vi "Data Logging Example.vi"() -> ()   [LabVIEW 2016]
panel:
  in  "File Name":string="log1.csv"
  in  "Header String":string="value 1, value 2, value 3"
  out "Line Written":bool=TRUE
  in  "Value 3":string="more than robots"
  in  "stop":bool
  in  "Logging Frequency":dbl(slide)=1.022434770467647 scale=0.1..20.0
  in  "Value 2":dbl(slide)=4.8979591836734695 scale=0.0..10.0
  in  "Value 1":dbl(slide)=2.3469387755102042 scale=0.0..10.0
  # "Set these controls before running the example"
  # "This example demonstrates how to write data to a file on the SD card of the Huskie Board.\n\nSpecify the file name and the header string before running the example. The file name must conform to \"8.3' file name conventions. That is there can be at most eight characters followed by a period followed by a three character extension.\n\nThe reminaing controls may be changed while the example is running. All values written to the log must be strings. This example shows how to convert numbers to strings before invoking the HB_WriteToLog VI.\n\nPlease note that only one file may be open at a time."
  # "Change these controls while running the example"
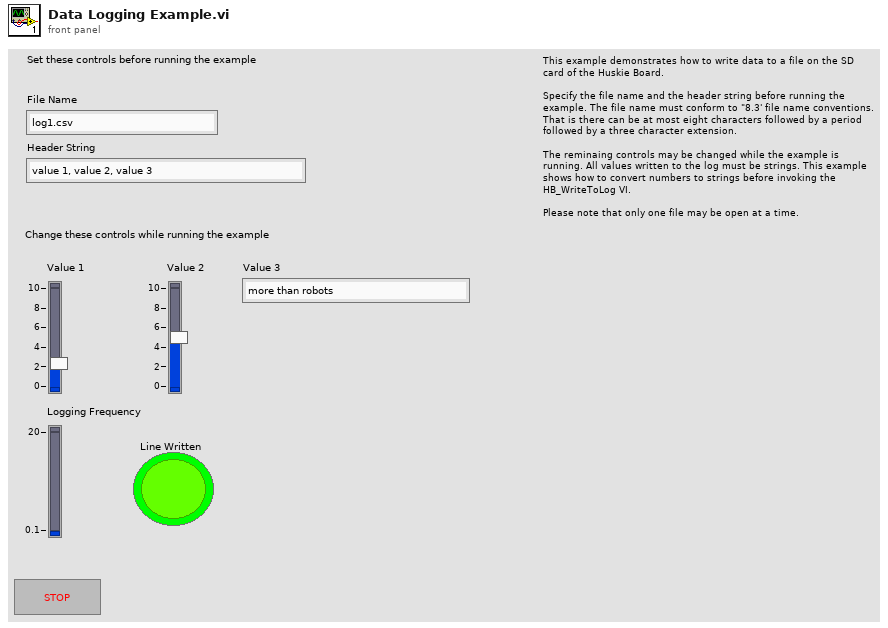
[diagram p1: front panel]
types:
  T1 = typedef "WPI_SerialPortRef.ctl" = cluster{"DevStatus":errorcluster, "Serial Port Name":refnum<visa-resource-name>}
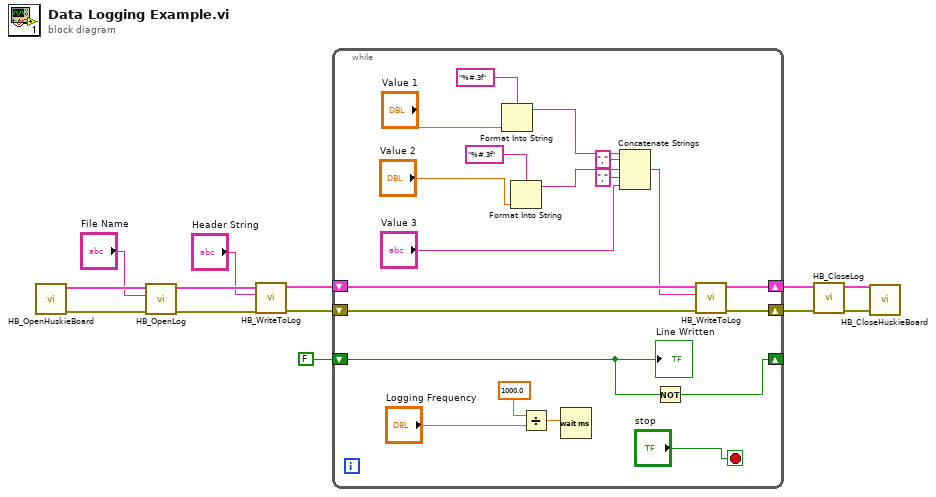
[diagram p0: block diagram]
diagram:
  n1 = call <vilib>:"HB_OpenHuskieBoard.vi"() -> ("error out"=w10:errorcluster, "HBDeviceRef"=w12:T1)  [unwired: 10 in]
  n2 = call <vilib>:"HB_OpenLog.vi"("error in (no error)"=w10, "File Name"="File Name", "HBDeviceRef"=w12) -> ("error out"=w9:errorcluster, "HBDeviceRef"=w6:T1)  [unwired: 7 in]
  n3 = call <vilib>:"HB_WriteToLog.vi"("error in (no error)"=w9, "Log string"="Header String", "HBDevRef"=w6) -> ("error out"=w8:errorcluster, "HBDevRef"=w7:T1)  [unwired: 7 in]
  n4 = while {
    shift-right: [w22] -> _
    shift-left: FALSE -> [w23]
    shift-right: [w17] -> w3
    shift-left: w7 -> [w16]
    shift-right: [w18] -> w4
    shift-left: w8 -> [w15]
    stop <- "stop" stop-if-true
    n5 = Format Into String(format string="%#.3f", "Value 1") -> (resulting string=w28:string)  [unwired: 2 in, 1 out]
    n6 = Format Into String(format string="%#.3f", "Value 2") -> (resulting string=w29:string)  [unwired: 2 in, 1 out]
    n7 = Divide(x=1000.0, y="Logging Frequency") -> (x/y=w21:dbl)
    n8 = Wait (ms)(milliseconds to wait=w21) -> ()  [unwired: 1 out]
    n9 = Concatenate Strings(w28, "," ("string"), w29, "," ("string"), "Value 3") -> (w14:string)
    n10 = Not(x=w23) -> (.not. x?=w22:bool)
    n11 = call <vilib>:"HB_WriteToLog.vi"("error in (no error)"=w15, "Log string"=w14, "HBDevRef"=w16) -> ("error out"=w18:errorcluster, "HBDevRef"=w17:T1)  [unwired: 7 in]
    "Line Written" <- w23
  }
  n12 = call <vilib>:"HB_CloseLog.vi"("error in (no error)"=w4, "HBDeviceRef"=w3) -> ("error out"=w1:errorcluster, "HBDeviceRef"=w2:T1)  [unwired: 8 in]
  n13 = call <vilib>:"HB_CloseHuskieBoard.vi"("error in (no error)"=w1, "HBDeviceRef"=w2) -> ()  [unwired: 9 in, 1 out]
